vi "FormatBoolean.vi"(1 "boolean":bool) -> (0 "value":string)   [LabVIEW 2014, in "Raspberry Pi Compatible Compiler for LabVIEW.lvlib" / "PythonConfiguration.lvclass"]
uses:
  PythonConfiguration.lvclass
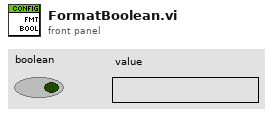
[diagram p1: front panel]
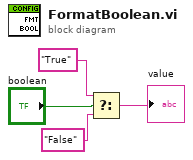
[diagram p0: block diagram]
diagram:
  n1 = Select(t="True" ("format string"), s="boolean", f="False" ("format string")) -> (s? t:f=→"value":string)
